vi "Read CCD Config.vi"(8 "error in (no error)":errorcluster, 11 "CCDCamera in":refnum<class "Sim_Ixon_Ultra.lvclass">) -> (0 "error out":errorcluster, 2 "CCD Config":T1, 3 "CCDCamera out":refnum<class "Sim_Ixon_Ultra.lvclass">)   [LabVIEW 2018, in "Sim_Ixon_Ultra.lvclass"]
uses:
  Sim_Ixon_Ultra.lvclass
  Sim_Ixon_Ultra.lvclass/Sim_Ixon_Ultra.ctl
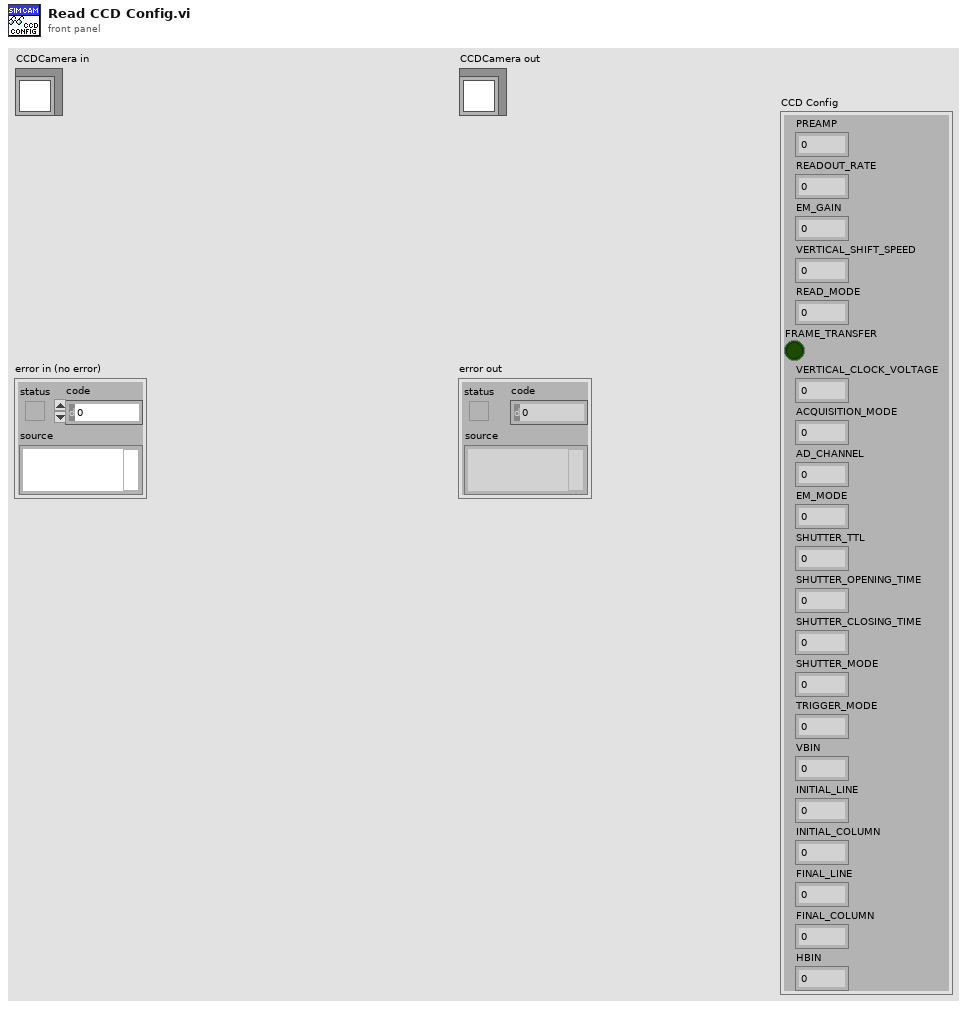
[diagram p1: front panel]
types:
  T1 = cluster{"PREAMP":u16, "READOUT_RATE":u16, "EM_GAIN":u16, "VERTICAL_SHIFT_SPEED":u16, "READ_MODE":u16, "FRAME_TRANSFER":bool, "VERTICAL_CLOCK_VOLTAGE":u16, "ACQUISITION_MODE":u16, "AD_CHANNEL":u16, "EM_MODE":u16, "SHUTTER_TTL":u16, "SHUTTER_OPENING_TIME":u16, "SHUTTER_CLOSING_TIME":u16, "SHUTTER_MODE":u16, "TRIGGER_MODE":u16, "VBIN":u16, "INITIAL_LINE":u16, "INITIAL_COLUMN":u16, "FINAL_LINE":u16, "FINAL_COLUMN":u16, "HBIN":u16}
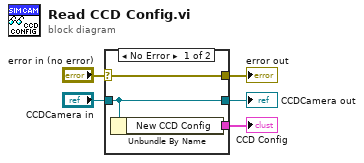
[diagram p0: block diagram]
diagram:
  n1 = case shown="No Error" "error in (no error)" {
    selector: "error in (no error)" -> [w7 w9]
    tunnel: [w7 w9] -> w4
    tunnel: [w8 w10] -> w2
    tunnel: "CCDCamera in" -> [w8 w10]
    tunnel: [w6 _] -> w1
    frame No Error {
      n2 = Unbundle By Name(w8) -> ("New CCD Config"=w6:T1)
    }
    frame Error {
    }
  }
  "error out" <- w4
  "CCDCamera out" <- w2
  "CCD Config" <- w1
